vi "Butterfly_PullUp Capacitance_ERMod.vi"(0 "Semiconductor Module Context":T2, 3 "C_TH_Delta":dbl=0.03 format="%#_13g", 4 "VNAs Measurement Parameters":T1, 5 "error in (no error)":errorcluster, 9 "Start_v":dbl=10.0 format="%#_13g", 11 "Stop_v":dbl=41.0 format="%#_13g") -> (14 "Semiconductor Module Context Out":T2, 19 "error out":errorcluster)   [LabVIEW 2013]
uses:
  <vilib>/NI_TestStand_SemiconductorModule/NI_TestStand_Semiconductor_Module.lvlibp/PinMap/General/SemiconductorModuleContext.ctl
  VNA/VNAs Measurement Parameters.ctl
  <instrlib>/niDCPower/nidcpower.llb/niDCPower Wait For Event - Event.ctl
  <vilib>/NI_TestStand_SemiconductorModule/NI_TestStand_Semiconductor_Module.lvlibp/PinMap/DC Power/PinToNIDCPowerSession.vi
  <vilib>/NI_TestStand_SemiconductorModule/NI_TestStand_Semiconductor_Module.lvlibp
  VNA/Pin Map API/VNA Custom Instrument.lvlib
  <vilib>/NI_TestStand_SemiconductorModule/NI_TestStand_Semiconductor_Module.lvlibp/PinMap/General/Publish/PublishDataDouble2D.vi
panel:
  in  "PU_Pin":string="SMU_PD"
  in  "RFPins":string[](array[string])
  out "Site":i32
  out "RL Step":i32
  out "PI Step":i32
  out "C_TH_PU":dbl format="%#_3g"
  out "C_Free":dbl[](array[numeric]) format="%#_3g"
  out "max index":i32
  out "BF C PI":dbl format="%#_3g"
  out "C_VPI":dbl
  out "BF C RL":dbl format="%#_3g"
  out "C_VRL":dbl
  out "appended array":dbl[][](array[numeric]) format="%#_3g"
  out "S3 steps":dbl[](array[numeric]) format="%#_3g"
  out "S2 steps":dbl[](array[numeric]) format="%#_3g"
  out "S1 steps":dbl[](array[numeric]) format="%#_3g"
  out "S0 steps":dbl[](array[numeric]) format="%#_3g"
  out "BF values":dbl[](array[numeric])
  out "VRLs":dbl[](array[numeric])
  out "VPIs":dbl[](array[numeric])
  out "Multisite Cap Data":dbl[][][](array[numeric])
  out "BF Names":string[](array[string])
  out "BFSamples":i32
  in  "Step_v":dbl=1.0
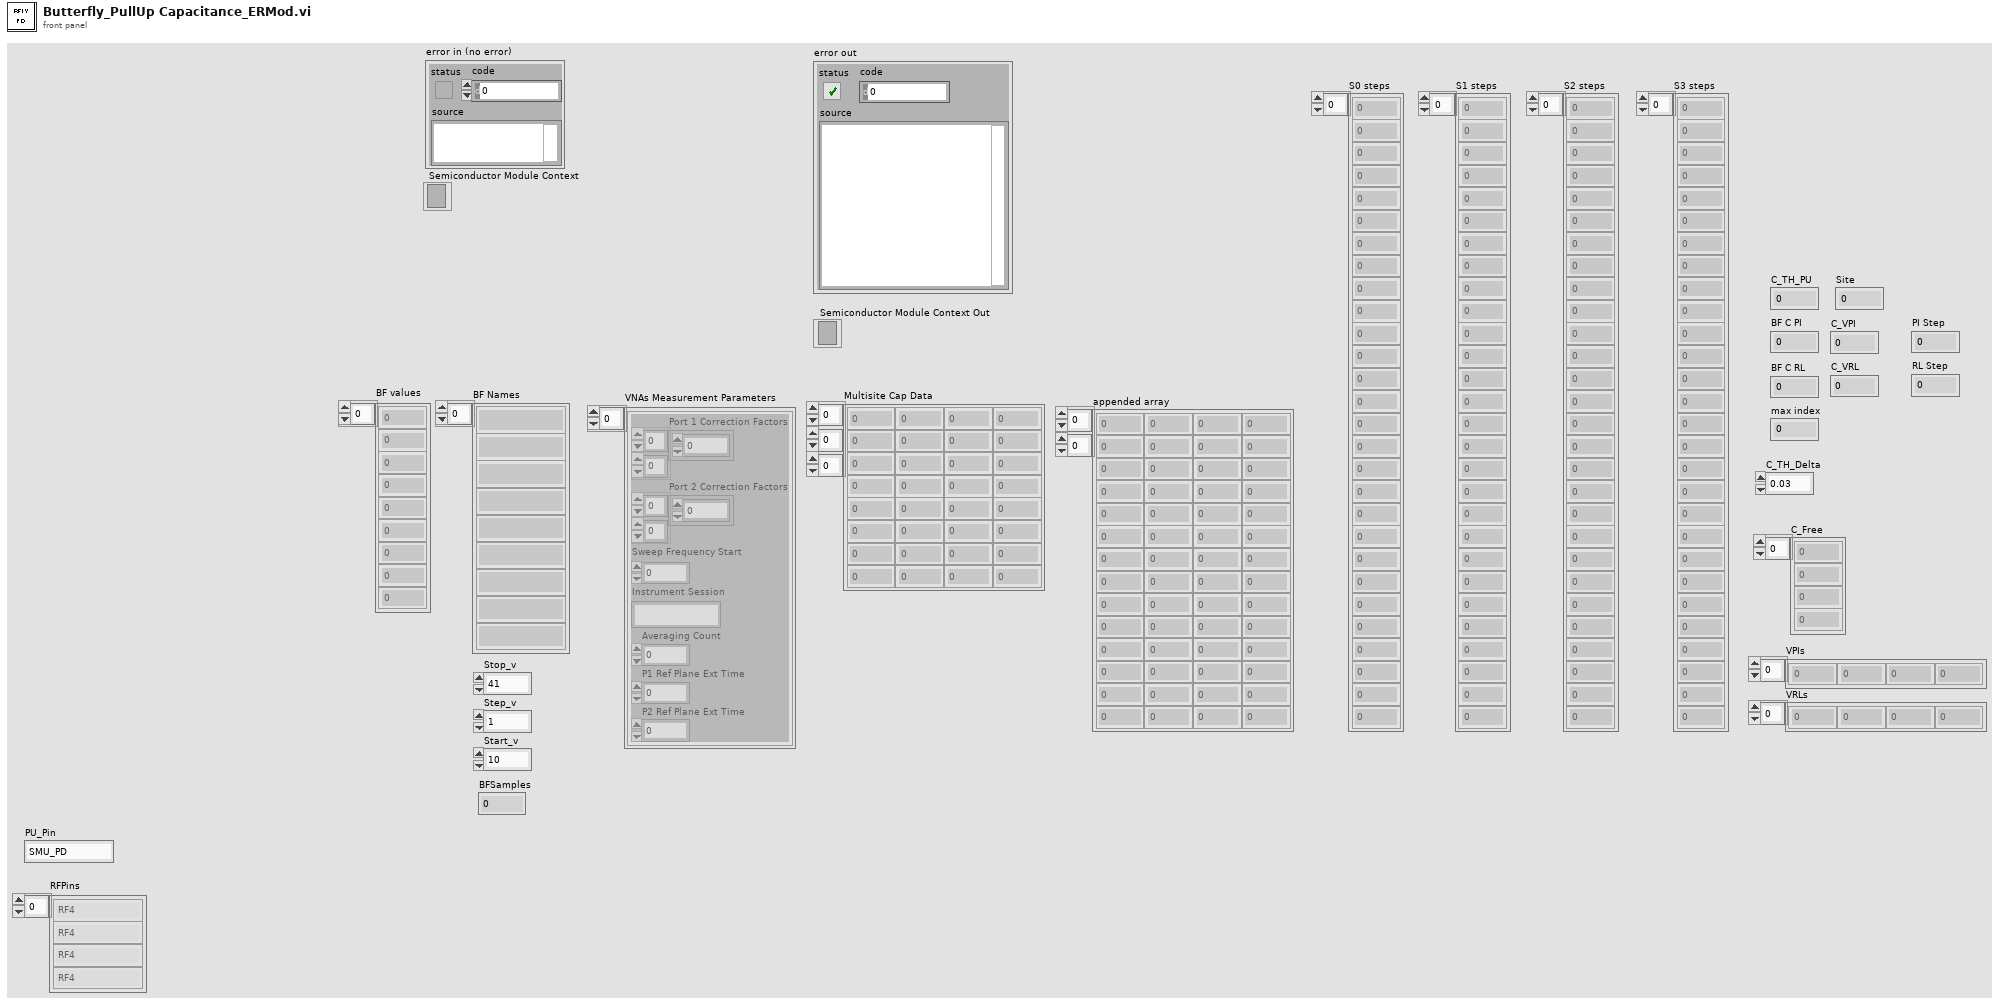
[diagram p1: front panel]
types:
  T1 = typedef "VNAs Measurement Parameters.ctl" = cluster{"Port 1 Correction Factors":cdb[][], "Port 2 Correction Factors":cdb[][], "Sweep Frequency Start":dbl, "Instrument Session":string, "Averaging Count":i32, "P1 Ref Plane Ext Time":dbl, "P2 Ref Plane Ext Time":dbl}[]
  T2 = typedef "NI_TestStand_Semiconductor_Module.lvlibp/SemiconductorModuleContext.ctl" = refnum<k7>
  T3 = typedef "niDCPower Wait For Event - Event.ctl" = i32
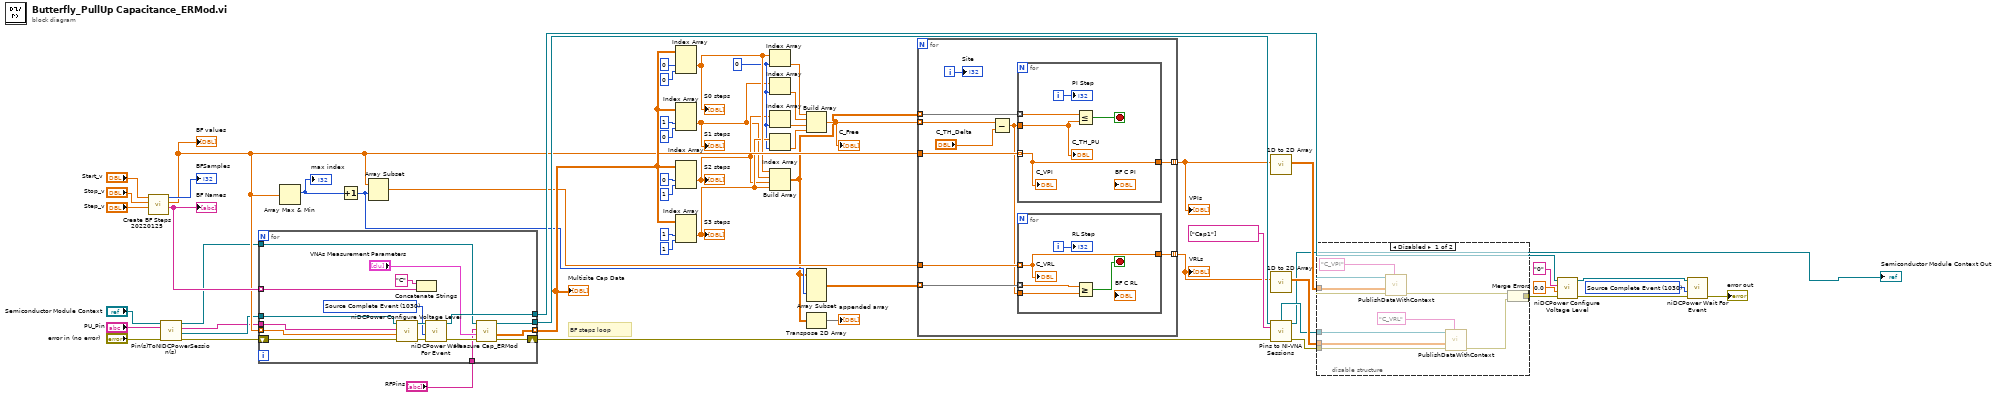
[diagram p0: block diagram]
diagram:
  w18 = 0 ("index")
  w46 = T3 1030 items=["Source Complete Event"=1030, "Measure Complete Event"=1031, "Sequence Iteration Complete Event"=1032, "Sequence Engine Done Event"=1033, "Pulse Complete Event"=1051, "Ready For Pulse Trigger Event"=1052] ("event")
  # "BF steps loop"
  n1 = call "Create BF Steps 20220125.vi"("Step_v"="Step_v", "Stop_v"="Stop_v", "Start_v"="Start_v") -> ("BF Names"=w52:string[], "BF values"=w25:dbl[], "BFSamples"=→"BFSamples":i32)  [unwired: 6 in]
  "BF Names" <- w52
  "BF values" <- w25
  n2 = call-poly <vilib>:"Pin(s)ToNIDCPowerSession(s).vi"("error in (no error)"="error in (no error)", "Pin"="PU_Pin", "Semiconductor Module Context"="Semiconductor Module Context") -> ("error out"=w10:errorcluster, "Instrument Session"=w7:refnum<k15>, "Channel List"=w6:string, "Semiconductor Module Context Out"=w5:T2)  [unwired: 4 in, 1 out]
  n3 = for {
    shift-right: [w64] -> w44
    shift-left: w10 -> [w69]
    tunnel: w5 -> [w61]
    tunnel: [w62] -> w57
    tunnel: [w63] -> w45 mode=indexing
    tunnel: w52 -> [w73] mode=indexing
    tunnel: w25 -> [w68] mode=indexing
    tunnel: w7 -> [w67]
    tunnel: [w66] -> w49
    tunnel: w6 -> [w59]
    tunnel: "RFPins" -> [w58]
    w71 = T3 1030 items=["Source Complete Event"=1030, "Measure Complete Event"=1031, "Sequence Iteration Complete Event"=1032, "Sequence Engine Done Event"=1033, "Pulse Complete Event"=1051, "Ready For Pulse Trigger Event"=1052] ("event")
    n4 = call <instrlib>:"niDCPower Configure Voltage Level.vi"("error in (no error)"=w69, "voltage level"=w68, "channel name"=w59, "instrument handle"=w67) -> ("error out"=w70:errorcluster, "instrument handle out"=w72:refnum<k15>)  [unwired: 6 in]
    n5 = Concatenate Strings("C" ("string"), w73) -> ()  [unwired: 1 out]
    n6 = call <instrlib>:"niDCPower Wait For Event.vi"("error in (no error)"=w70, "event"=w71, "instrument handle"=w72) -> ("error out"=w60:errorcluster, "instrument handle out"=w66:refnum<k15>)  [unwired: 7 in]
    n7 = call "Measure Cap_ERMod.vi"("error in (no error)"=w60, "VNAs Measurement Parameters"="VNAs Measurement Parameters", "Pins"=w58, "Semiconductor Module Context"=w61) -> ("error out"=w64:errorcluster, "Multisite Cap Data"=w63:dbl[][], "Semiconductor Module Context Out"=w62:T2)  [unwired: 5 in]
  }
  "Multisite Cap Data" <- w45
  n8 = Array Max & Min(array=w25) -> (max index (indices)=w27:i32)  [unwired: 3 out]
  "max index" <- w27
  n9 = Increment(x=w27) -> (x+1=w26:i32)
  n10 = Array Subset(array=w25, index=w26) -> (w24:dbl[])  [unwired: 1 in]
  n11 = Index Array(array=w45, index (dim 1)=0 ("disabled index (row)"), index (dim 2)=0 ("disabled index (col)")) -> (element=w21:dbl[])  [unwired: 1 in]
  "S0 steps" <- w21
  n12 = Index Array(array=w45, index (dim 1)=1 ("index (row)"), index (dim 2)=0 ("index (col)")) -> (element=w12:dbl[])  [unwired: 1 in]
  "S1 steps" <- w12
  n13 = Index Array(array=w45, index (dim 1)=0 ("index (row)"), index (dim 2)=1 ("index (col)")) -> (element=w13:dbl[])  [unwired: 1 in]
  "S2 steps" <- w13
  n14 = Index Array(array=w45, index (dim 1)=1 ("index (row)"), index (dim 2)=1 ("index (col)")) -> (element=w19:dbl[])  [unwired: 1 in]
  "S3 steps" <- w19
  n15 = Index Array(array=w21, index=w18) -> (element=w20:dbl)
  n16 = Index Array(array=w12, index=w18) -> (element=w17:dbl)
  n17 = Index Array(array=w13, index=w18) -> (element=w15:dbl)
  n18 = Index Array(array=w19, index=w18) -> (element=w16:dbl)
  n19 = Build Array(w21, w12, w13, w19) -> (w11:dbl[][])
  n20 = Build Array(w20, w17, w15, w16) -> (w14:dbl[])
  "C_Free" <- w14
  n21 = Array Subset(array=w11, index (col)=w26) -> (w28:dbl[][])  [unwired: 3 in]
  n22 = Transpose 2D Array(2D array=w11) -> (transposed array=→"appended array":dbl[][])
  n23 = for {
    tunnel: w25 -> [w84]
    tunnel: [w83] -> w23 mode=indexing
    tunnel: w24 -> [w82]
    tunnel: w28 -> [w81] mode=indexing
    tunnel: [w80] -> w22 mode=indexing
    tunnel: w14 -> [w77] mode=indexing
    tunnel: w11 -> [w78] mode=indexing
    i -> [w79]
    n24 = Subtract(x=w77, y="C_TH_Delta") -> (x-y=w75:dbl)
    n25 = for {
      tunnel: w84 -> [w93] mode=indexing
      tunnel: [w93] -> w83
      tunnel: w75 -> [w92]
      tunnel: w78 -> [w90] mode=indexing
      i -> [w91]
      stop <- w94 stop-if-true
      n26 = Less Or Equal?(x=w90, y=w92) -> (x <= y?=w94:bool)
      "C_VPI" <- w93
      "C_TH_PU" <- w92
      "PI Step" <- w91
    }
    n27 = for {
      tunnel: w82 -> [w88] mode=indexing
      tunnel: w81 -> [w85] mode=indexing
      tunnel: [w88] -> w80
      tunnel: w75 -> [w87]
      i -> [w86]
      stop <- w89 stop-if-true
      n28 = Greater Or Equal?(x=w85, y=w87) -> (x >= y?=w89:bool)
      "C_VRL" <- w88
      "RL Step" <- w86
    }
    "Site" <- w79
  }
  "VPIs" <- w23
  "VRLs" <- w22
  n29 = call "1D to 2D Array.vi"("1D Array"=w23) -> ("2D Array"=w30:dbl[][])  [unwired: 10 in]
  n30 = call "1D to 2D Array.vi"("1D Array"=w22) -> ("2D Array"=w42:dbl[][])  [unwired: 10 in]
  n31 = call "Pins to NI-VNA Sessions.vi"("Semiconductor Module Context"=w57, "Pins"=string[] ["Cap1"] ("Capacitance Pins"), "error in (no error)"=w44) -> ("Pin Query Context"=w31:refnum<class "MultiplePinMultipleSessionQueryContext.lvclass">, "Semiconductor Module Context Out"=→"Semiconductor Module Context Out":T2, "error out"=w29:errorcluster)  [unwired: 8 in, 2 out]
  n32 = disable-structure shown="Disabled" {
    disable-tunnel: [w103 w104] -> w43
    disable-tunnel: w42 -> [w101 _]
    disable-tunnel: w31 -> [w99 _]
    disable-tunnel: w30 -> [w98 _]
    disable-tunnel: w29 -> [w95 w104]
    frame Disabled {
      n33 = call-poly <vilib>:"PublishDataWithContext.vi"("Published Data Id"="C_VPI", "error in (no error)"=w95, "Data In"=w98, "Pin Query Context"=w99) -> ("error out"=w96:errorcluster)  [unwired: 6 in, 1 out]
      n34 = call-poly <vilib>:"PublishDataWithContext.vi"("Published Data Id"="C_VRL", "error in (no error)"=w95, "Data In"=w101, "Pin Query Context"=w99) -> ("error out"=w102:errorcluster)  [unwired: 6 in, 1 out]
      n35 = Merge Errors(w96, w102) -> (w103:errorcluster)
    }
    frame Enabled {
    }
  }
  n36 = call <instrlib>:"niDCPower Configure Voltage Level.vi"("error in (no error)"=w43, "voltage level"=0.0, "channel name"="0", "instrument handle"=w49) -> ("error out"=w48:errorcluster, "instrument handle out"=w47:refnum<k15>)  [unwired: 6 in]
  n37 = call <instrlib>:"niDCPower Wait For Event.vi"("error in (no error)"=w48, "event"=w46, "instrument handle"=w47) -> ("error out"=→"error out":errorcluster)  [unwired: 7 in, 1 out]
